vi "addChangeVectors.vi"(4 "keySettings":T1 {"clipPercentile" min=0.0 max=100.0 step=0.1 format="%#_g%%"}, 6 "vectorDims":cluster{"vectorSize":sgl, "vectorScale":dbl}={"vectorSize"=3.0, "vectorScale"=5.0}, 7 "channelValues":string[][](array[string]), 8 "error in (no error)":errorcluster, 9 "Multi Ordinate":i32[](array[numeric]), 10 "Plotted Series":bool[][](array[boolean]), 11 "parentObjectIn":refnum<vi>) -> (0 "error out":errorcluster, 1 "colourRampVals":cluster{"value":dbl, "colour":u32}[](array[cluster]), 2 "STLs":cluster{"coordSys":T2, "WD":dbl, "STL":string}[](array[cluster]), 3 "parentObjectOut":refnum<vi>, 5 "whitePoint":dbl format="%0.2f")   [LabVIEW 2022 SP3]
uses:
  coordSys.ctl
  c96bb956-68e0-db40-bc82-d68bd366085b.vi
  06b26dab-0252-3542-972b-6a5dd2eb14e0.vi
  eb984068-d2c5-9543-b0d0-bd690a949330.vi
  e414c31b-eb45-3c41-805f-0ddbe17f6227.vi
  253da183-7414-e34d-8f16-197921a1110c.vi
  <vilib>/picture/3D Picture Control/Object/Create Object (name).vi
  <vilib>/picture/3D Picture Control/Object/Add Object (reference).vi
  <vilib>/picture/3D Picture Control/NI_3D Picture Control.lvlib
panel:
  out "notRefnum":bool
  out "Name":string
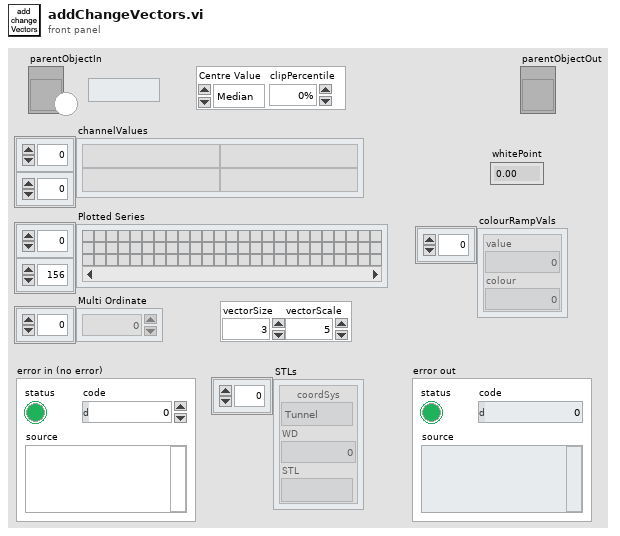
[diagram p1: front panel]
types:
  T1 = cluster{"Centre Value":enum16{"Median", "Zero"}, "clipPercentile":dbl}
  T2 = typedef "coordSys.ctl" = enum16{"Tunnel", "Model"}
  T3 = enum16{"Overall Median", "Baseline Median", "Zero"}
  T4 = typedef "vectorDef.ctl" = cluster{"pointID":string[], "XYZ-WD":dbl[][], "UVW-TI":dbl[][], "CoordSys":T2[]}
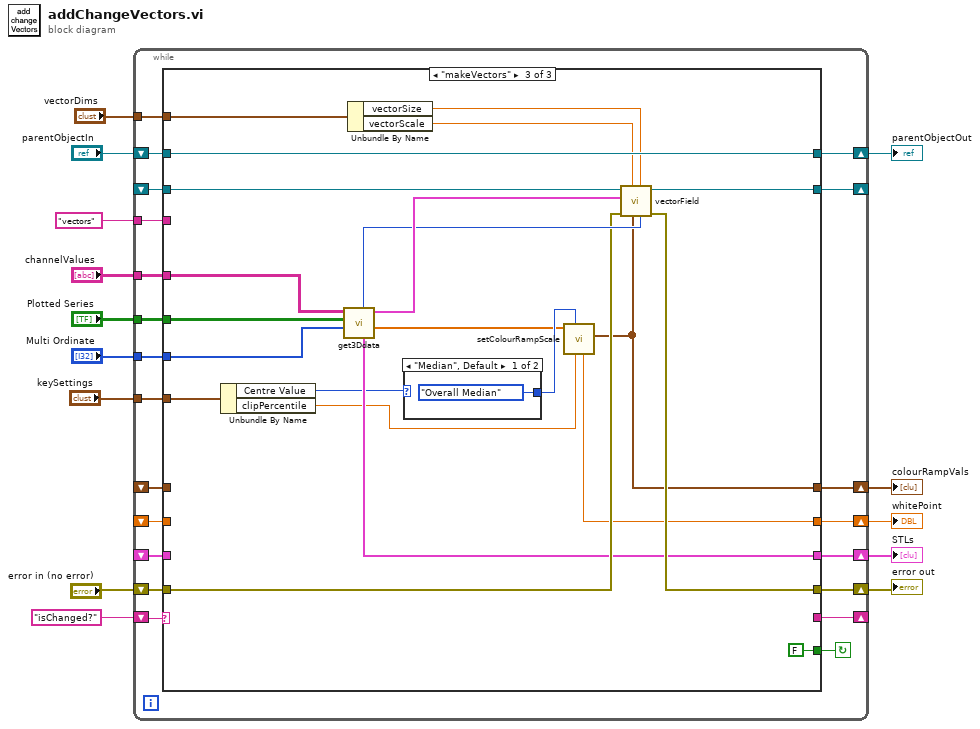
[diagram p0: block diagram]
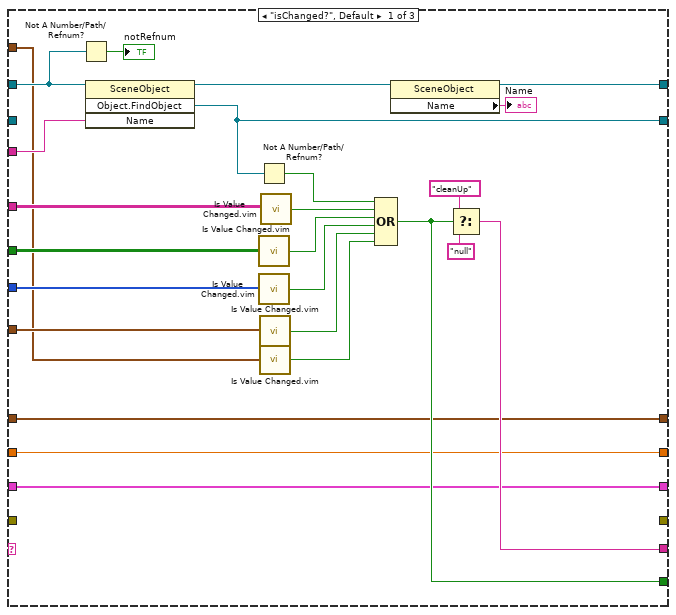
[diagram p2: hidden frame]
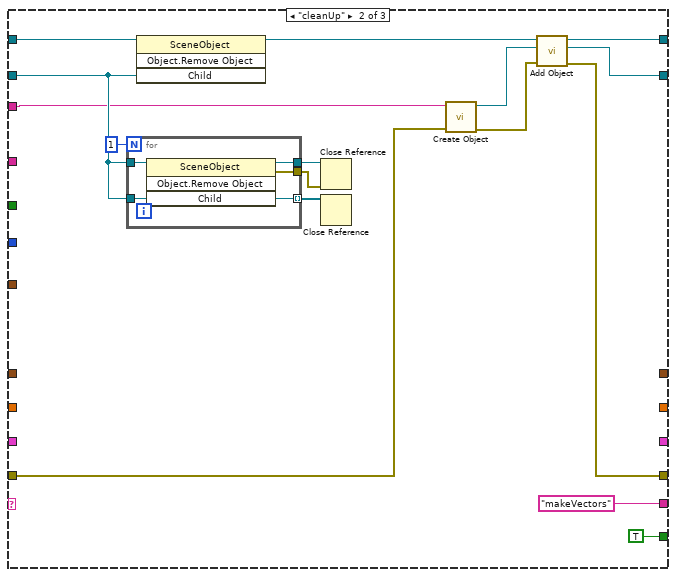
[diagram p3: hidden frame]
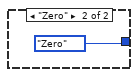
[diagram p4: hidden frame]
diagram:
  n1 = while {
    shift-right: [w34] -> w13
    shift-left: "parentObjectIn" -> [w35]
    shift-right: [w33] -> _
    shift-left: _ -> [w25]
    tunnel: "vectors" ("Name") -> [w32]
    tunnel: "channelValues" -> [w31]
    tunnel: "Plotted Series" -> [w30]
    tunnel: "Multi Ordinate" -> [w29]
    shift-right: [w28] -> _
    shift-left: "isChanged?" ("t") -> [w27]
    shift-right: [w24] -> w6
    shift-left: "error in (no error)" -> [w23]
    tunnel: "keySettings" -> [w22]
    tunnel: "vectorDims" -> [w21]
    shift-right: [w20] -> w3
    shift-left: _ -> [w19]
    shift-right: [w17] -> w1
    shift-left: _ -> [w16]
    shift-right: [w18] -> w2
    shift-left: _ -> [w15]
    stop <- w26 continue-if-true
    n2 = case shown="\"makeVectors\"" w27 {
      tunnel: w35 -> [w57 w74 w100]
      tunnel: [w56 w68 w100] -> w34
      tunnel: [w50 w67 w82] -> w33
      tunnel: w32 -> [w49 w65 _]
      tunnel: w31 -> [w48 _ w98]
      tunnel: w30 -> [w47 _ w97]
      tunnel: w29 -> [w46 _ w96]
      tunnel: [w44 "makeVectors" ("t") _] -> w28
      tunnel: [w43 TRUE FALSE] -> w26
      tunnel: w25 -> [_ w70 w81]
      tunnel: [_ w62 w91] -> w24
      tunnel: w23 -> [_ w64 w95]
      tunnel: w22 -> [w42 _ w94]
      tunnel: w21 -> [w41 _ w90]
      tunnel: [w38 _ w89] -> w20
      tunnel: w19 -> [w38 _ _]
      tunnel: [w36 _ w84] -> w18
      tunnel: [w37 _ w83] -> w17
      tunnel: w16 -> [w37 _ _]
      tunnel: w15 -> [w36 _ _]
      frame "isChanged?", Default {
        n3 = Not A Number/Path/Refnum?(number/path/refnum=w57) -> (NaN/Path/Refnum?=→"notRefnum":bool)
        n4 = invoke class="SceneObject" method="Object.FindObject"(reference=w57, "Name"=w49) -> (reference out=w59:refnum<vi>, "FindObject"=w50:refnum<vi>)  [unwired: 2 in, 2 out]
        n5 = Not A Number/Path/Refnum?(number/path/refnum=w50) -> (NaN/Path/Refnum?=w54:bool)
        n6 = call "Is Value Changed.vim"("value"=w47) -> ("changed or first call?"=w52:bool)
        n7 = call "Is Value Changed.vim"("value"=w46) -> ("changed or first call?"=w45:bool)
        n8 = call "Is Value Changed.vim"("value"=w42) -> ("changed or first call?"=w40:bool)
        n9 = call "Is Value Changed.vim"("value"=w41) -> ("changed or first call?"=w39:bool)
        n10 = call "Is Value Changed.vim"("value"=w48) -> ("changed or first call?"=w51:bool)
        n11 = Compound Arithmetic op=OR(w54, w51, w52, w45, w40, w39) -> (w43:bool)
        n12 = property class="SceneObject"(reference=w59) -> (reference out=w56:refnum<vi>, "Name"=→"Name":string)  [unwired: 1 in, 1 out]
        n13 = Select(t="cleanUp", s=w43, f="null") -> (s? t:f=w44:string)
      }
      frame "cleanUp" {
        n14 = for {
          N: 1 -> [_]
          tunnel: w70 -> [w80]
          tunnel: [w79] -> w75
          tunnel: [w78] -> w76
          tunnel: [w77] -> w71 mode=indexing
          tunnel: w70 -> [w77]
          n15 = invoke class="SceneObject" method="Object.Remove Object"(reference=w80, "Child"=w77) -> (reference out=w79:refnum<vi>, error out=w78:errorcluster)  [unwired: 2 in, 2 out]
        }
        n16 = invoke class="SceneObject" method="Object.Remove Object"(reference=w74, "Child"=w70) -> (reference out=w69:refnum<vi>)  [unwired: 2 in, 3 out]
        n17 = Close Reference(reference=w75, error in (no error)=w76) -> ()  [unwired: 1 out]
        n18 = Close Reference(reference=w71) -> ()  [unwired: 1 in, 1 out]
        n19 = call-poly <vilib>:"Create Object.vi"("error in (no error)"=w64, "Name"=w65) -> ("error out"=w63:errorcluster, "Scene:New Object"=w66:refnum<vi>)  [unwired: 8 in]
        n20 = call-poly <vilib>:"Add Object.vi"("error in (no error)"=w63, "New Object In"=w66, "Scene Object In"=w69) -> ("error out"=w62:errorcluster, "New Object Out"=w67:refnum<vi>, "Scene Object Out"=w68:refnum<vi>)  [unwired: 6 in]
      }
      frame "makeVectors" {
        n21 = Unbundle By Name(w94) -> ("Centre Value"=w87:enum16{"Median", "Zero"}, "clipPercentile"=w85:dbl)
        n22 = call "get3Ddata.vi"("plottedVariables"=w96, "Plotted Series"=w97, "allTheData"=w98) -> ("scalarVals"=w86:dbl[], "vectorInfo"=w102:T4, "STLs"=w89:cluster{"coordSys":T2, "WD":dbl, "STL":string}[], "mostCoords"=w101:T2)  [unwired: 5 in]
        n23 = Unbundle By Name(w90) -> ("vectorSize"=w93:sgl, "vectorScale"=w92:dbl)
        n24 = case shown="\"Median\", Default" w87 {
          tunnel: [T3."Overall Median" ("Centre Value") T3."Zero" ("Centre Value")] -> w88
          frame "Median", Default {
          }
          frame "Zero" {
          }
        }
        n25 = call "setColourRampScale.vi"("scaleClipPercentile"=w85, "Centre Value"=w88, "baselineData"=w86) -> ("colourRampVals"=w83:cluster{"value":dbl, "colour":u32}[], "whitePoint"=w84:dbl)  [unwired: 7 in]
        n26 = call "vectorField.vi"("mostCoords"=w101, "thiccness"=w93, "colourRampVals"=w83, "scale"=w92, "error in (no error)"=w95, "vectorInfo"=w102, "SceneObject in"=w81) -> ("error out"=w91:errorcluster, "SceneObject out"=w82:refnum<vi>)  [unwired: 3 in]
      }
    }
  }
  "error out" <- w6
  "parentObjectOut" <- w13
  "STLs" <- w3
  "whitePoint" <- w2
  "colourRampVals" <- w1
